vi "Create All Host Message Queues.vi"(8 "error in (no error)":errorcluster) -> (0 "error out":errorcluster, 3 "Message Queues out":T1)   [LabVIEW 2017, in "Message Queue.lvlib"]
doc: "This VI creates and initializes all the message queues for your application. If your application requires more than one message queue, right-click the \"Message Queues\" constant above and select Open Type Def. Add the new Message Queue(s) to the type definition, then initialize them in this VI."
uses:
  Message Queue.lvlib
  All Host Message Queues.ctl
  Message Cluster.ctl
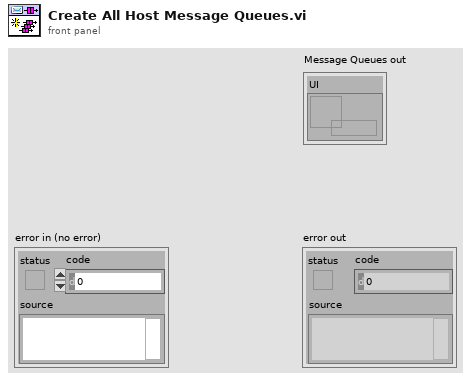
[diagram p1: front panel]
types:
  T1 = typedef "Message Queue.lvlib/All Host Message Queues.ctl" = cluster{"UI":refnum<queue>}
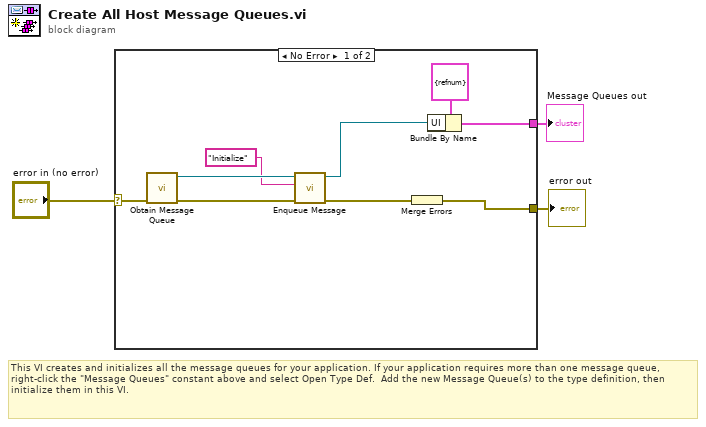
[diagram p0: block diagram]
diagram:
  # "This VI creates and initializes all the message queues for your application. If your application requires more than one message queue, right-click the \"Message Queues\" constant above and select Open Type Def.  Add the new Message Queue(s) to the type definition, then initialize them in this VI."
  n1 = case shown="No Error" "error in (no error)" {
    selector: "error in (no error)" -> [w7 w13]
    tunnel: [w4 w13] -> w3
    tunnel: [w10 _] -> w2
    frame No Error {
      n2 = call "Obtain Message Queue.vi"("error in (no error)"=w7) -> ("error out"=w9:errorcluster, "Message Queue"=w8:refnum<queue>)  [unwired: 9 in]
      n3 = call "Enqueue Message.vi"("error in (no error)"=w9, "Message"="Initialize", "Message Queue"=w8) -> ("error out"=w12:errorcluster, "dup Message Queue"=w5:refnum<queue>)  [unwired: 7 in]
      n4 = Merge Errors(w12) -> (w4:errorcluster)
      n5 = Bundle By Name(cluster=T1 {"UI"=refnum} ("Message Queues"), "UI"=w5) -> (w10:T1)
    }
    frame Error {
    }
  }
  "Message Queues out" <- w2
  "error out" <- w3
